vi "Initialize Oauth for QBO.vi"(6 "Refresh Token":string, 8 "Account ID":string, 9 "QBO Access Scope":T1, 10 "Client Secret":string, 11 "Client ID":string) -> (0 "error out":errorcluster, 3 "Oauth2.QBO":refnum<class "Oauth2.QBO.lvclass">)   [LabVIEW 2013, in "Oauth2.QBO.lvclass"]
uses:
  Oauth2.QBO.lvclass
  QBO Access Scopes.ctl
  Oauth2/Oauth2.lvclass
  <vilib>/LabVIEW Open Source Project/Data Manipulation/Variant/OpenVariant.lvlib
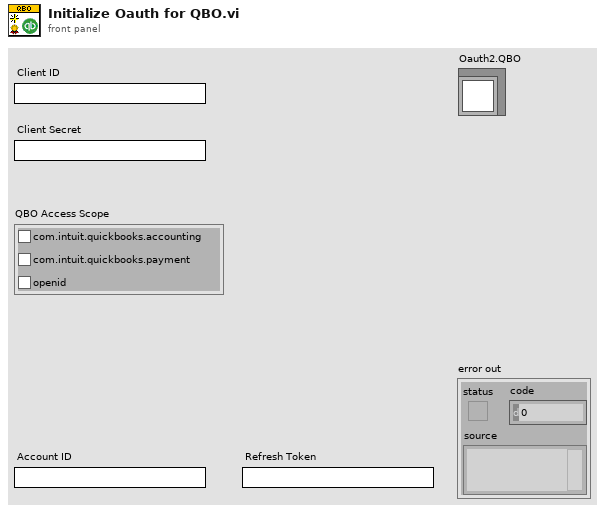
[diagram p1: front panel]
types:
  T1 = typedef "Oauth2.QBO.lvclass/QBO Access Scopes.ctl" = cluster{"com.intuit.quickbooks.accounting\t":bool, "com.intuit.quickbooks.payment\t":bool, "openid\t":bool}
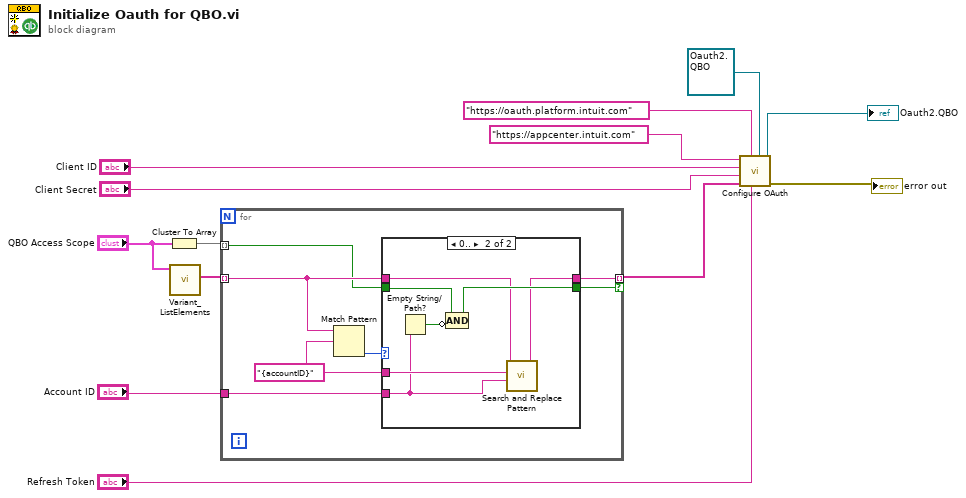
[diagram p0: block diagram]
diagram:
  n1 = Cluster To Array(cluster="QBO Access Scope") -> (array=w12:bool[])
  n2 = call <vilib>:"Variant_ListElements.vi"("Variant"="QBO Access Scope") -> ("element names"=w13:string[])  [unwired: 7 in, 3 out]
  n3 = for {
    tunnel: [w18] -> w11 mode=indexing if=w17
    tunnel: w13 -> [w19] mode=indexing
    tunnel: w12 -> [w16] mode=indexing
    tunnel: "Account ID" -> [w15]
    w14 = "{accountID}" ("regular expression")
    n4 = Match Pattern(string=w19, regular expression=w14) -> (offset past match=w20:i32)  [unwired: 1 in, 3 out]
    n5 = case shown="0.." w20 {
      tunnel: w19 -> [w22 w26]
      tunnel: [w22 w25] -> w18
      tunnel: [w21 w27] -> w17
      tunnel: w16 -> [w21 w28]
      tunnel: w15 -> [_ w23]
      tunnel: w14 -> [_ w24]
      frame Default {
      }
      frame 0.. {
        n6 = Empty String/Path?(string/path=w23) -> (empty?=w29:bool)
        n7 = Compound Arithmetic op=AND(w28, invert w29) -> (w27:bool)
        n8 = call <vilib>:"Search and Replace Pattern.vi"("string"=w26, "regular expression (\"\")"=w24, "replace string (\"\")"=w23) -> ("result string"=w25:string)  [unwired: 2 in, 1 out]
      }
    }
  }
  n9 = call "Configure OAuth.vi"("Oauth2 in"=refnum<class "Oauth2.QBO.lvclass"> refnum ("Oauth2.Harvest in"), "Refresh Token"="Refresh Token", "Exchange Code Server URI"="https://oauth.platform.intuit.com" ("path"), "scopes"=w11, "Client Secret"="Client Secret", "Client ID"="Client ID", "Authorization Server URI"="https://appcenter.intuit.com" ("path")) -> ("error out"=→"error out":errorcluster, "Oauth2"=→"Oauth2.QBO":refnum<class "Oauth2.QBO.lvclass">)  [unwired: 3 in]
